vi "interfaceLoop idleStateCheck.vi"(7 "laserRefnum":refnum<vi>, 8 "error in (no error)":errorcluster, 9 "connectStateRefnum":refnum<data-value>, 11 "Stop":refnum<vi>) -> (0 "error out":errorcluster)   [LabVIEW 2018]
uses:
  PublicSubVI/Ctl/RegistyFunc.ctl
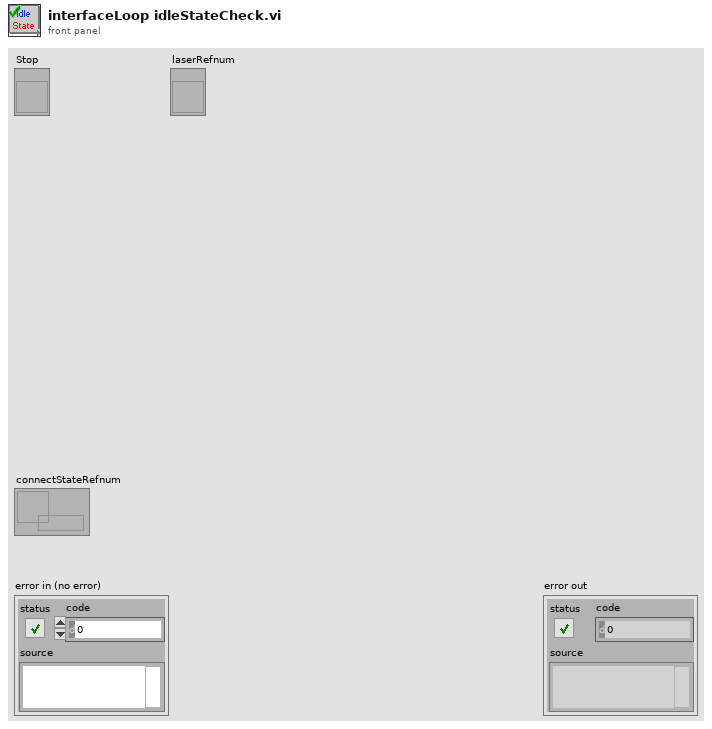
[diagram p1: front panel]
types:
  T1 = typedef "RegistyFunc.ctl" = enum16{"None", "FileAutoSave", "FileNoise", "FileSN", "ExeStatu", "WorkFolderPath", "MethodPath", "AVGItem", "LoopItem", "AutoRun", "BGColor", "LineColor", "LineWidth", "XGrid", "YGrid", "DeviceRefnum"}
  T2 = enum16{"init", "writeState", "readState", "close"}
  T3 = enum8{"Enabled", "Disabled", "Disabled and Grayed Out"}
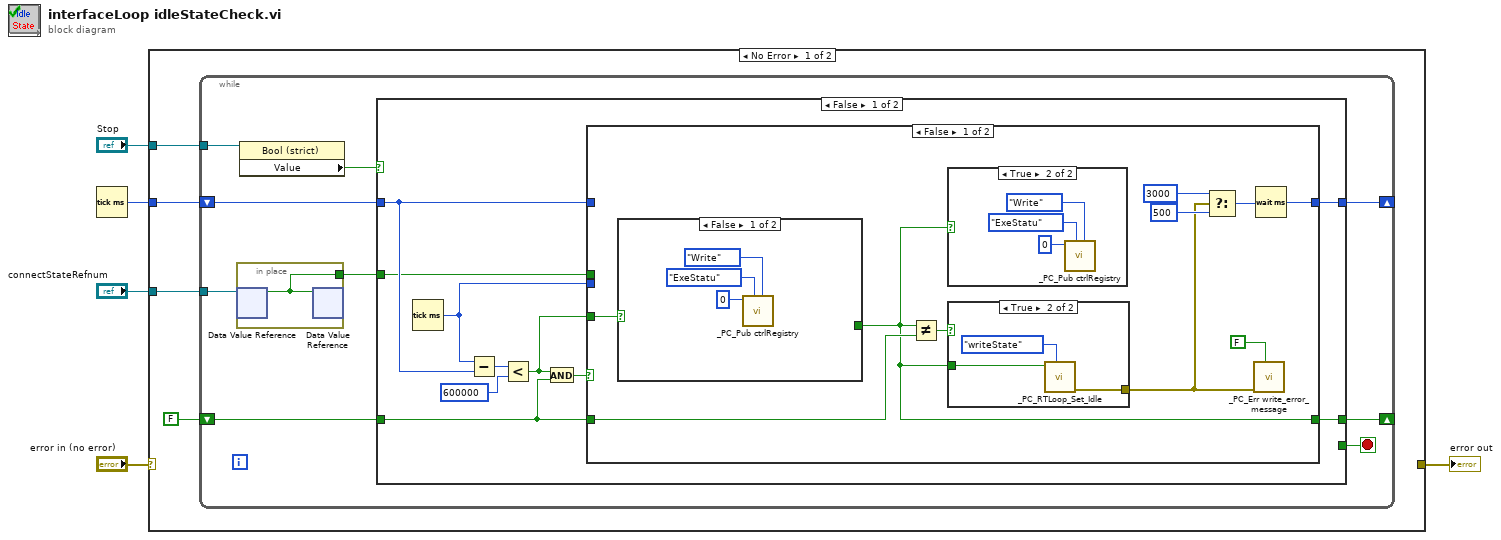
[diagram p0: block diagram]
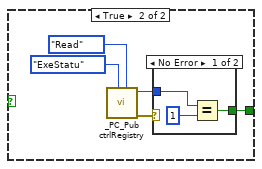
[diagram p2: hidden frame]
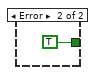
[diagram p3: hidden frame]
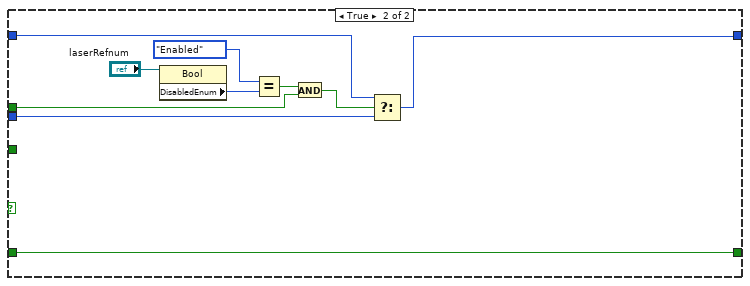
[diagram p6: hidden frame]
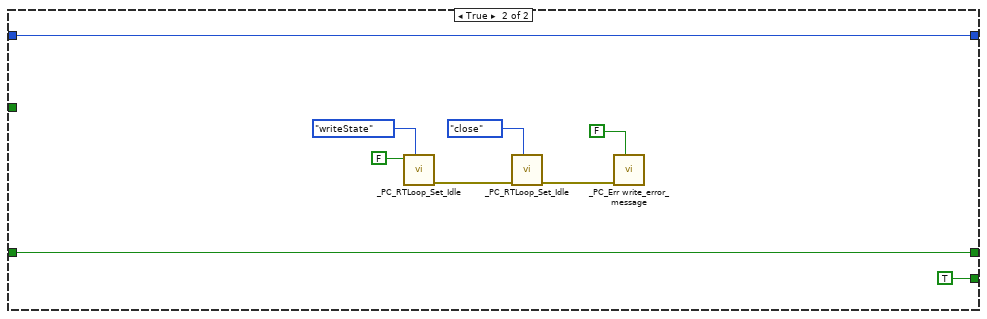
[diagram p7: hidden frame]
diagram:
  n1 = Tick Count (ms)() -> (millisecond timer value=w2:u32)
  n2 = case shown="No Error" "error in (no error)" {
    selector: "error in (no error)" -> [_ w77]
    tunnel: [_ w77] -> w4
    tunnel: "Stop" -> [w8 _]
    tunnel: w2 -> [w7 _]
    tunnel: "connectStateRefnum" -> [w6 _]
    frame No Error {
      n3 = while {
        tunnel: w8 -> [w18]
        shift-right: [w12] -> _
        shift-left: FALSE -> [w14]
        shift-right: [w13] -> _
        shift-left: w7 -> [w15]
        tunnel: w6 -> [w11]
        stop <- w16 stop-if-true
        n4 = in-place {
          in-place-border: [w19] -> w10
          n5 = in-place-dvr #1(w11) -> (w19:bool)  [unwired: 1 out]
          n6 = in-place-dvr #1(w19) -> ()  [unwired: 2 out]
        }
        n7 = property class="Bool (strict)"(reference=w18) -> ("Value"=w17:bool)  [unwired: 1 in, 2 out]
        n8 = case shown="False" w17 {
          tunnel: [_ TRUE] -> w16
          tunnel: w15 -> [w26 w75]
          tunnel: w14 -> [w24 w72]
          tunnel: [w25 w75] -> w13
          tunnel: [w23 w72] -> w12
          tunnel: w10 -> [w21 _]
          frame False {
            n9 = Tick Count (ms)() -> (millisecond timer value=w20:u32)
            n10 = Subtract(x=w20, y=w26) -> (x-y=w29:u32)
            n11 = Less?(x=w29, y=u32 600000) -> (x < y?=w22:bool)
            n12 = And(x=w22, y=w24) -> (x .and. y?=w27:bool)
            n13 = case shown="False" w27 {
              tunnel: w26 -> [_ w66]
              tunnel: [w36 w64] -> w25
              tunnel: w24 -> [w39 w67]
              tunnel: [w37 w67] -> w23
              tunnel: w22 -> [w35 _]
              tunnel: w21 -> [_ w59]
              tunnel: w20 -> [_ w65]
              frame False {
                n14 = case shown="False" w35 {
                  tunnel: [_ w43] -> w37
                  frame False {
                    n15 = call "_PC_Pub ctrlRegistry.vi"("type"=enum16{"None", "Write", "Read"}."Write", "function"=RegistyFunc."ExeStatu", "write value"=u32 0 ("y")) -> ()  [unwired: 5 in, 4 out]
                  }
                  frame True {
                    n16 = call "_PC_Pub ctrlRegistry.vi"("type"=enum16{"None", "Write", "Read"}."Read", "function"=RegistyFunc."ExeStatu") -> ("error out"=w45:errorcluster, "DWORD outpur"=w44:u32)  [unwired: 6 in, 2 out]
                    n17 = case shown="No Error" w45 {
                      tunnel: w44 -> [w50 _]
                      tunnel: [w48 TRUE] -> w43
                      frame No Error {
                        n18 = Equal?(x=w50, y=u32 1) -> (x = y?=w48:bool)
                      }
                      frame Error {
                      }
                    }
                  }
                }
                n19 = Not Equal?(x=w37, y=w39) -> (x != y?=w38:bool)
                n20 = case shown="True" w37 {
                  frame False {
                  }
                  frame True {
                    n21 = call "_PC_Pub ctrlRegistry.vi"("type"=enum16{"None", "Write", "Read"}."Write", "function"=RegistyFunc."ExeStatu", "write value"=u32 0 ("y")) -> ()  [unwired: 5 in, 4 out]
                  }
                }
                n22 = case shown="True" w38 {
                  tunnel: w37 -> [_ w57]
                  tunnel: [_ w55] -> w30
                  frame False {
                  }
                  frame True {
                    n23 = call "_PC_RTLoop_Set_Idle.vi"("Function"=T2."writeState", "exe_state"=w57) -> ("error out"=w55:errorcluster)  [unwired: 8 in, 1 out]
                  }
                }
                n24 = Select(t=u32 3000, s=w30, f=u32 500 ("milliseconds to wait")) -> (s? t:f=w32:u32)
                n25 = call "_PC_Err write_error_message.vi"("show msg( T )"=FALSE, "error in"=w30) -> ()  [unwired: 9 in, 1 out]
                n26 = Wait (ms)(milliseconds to wait=w32) -> (millisecond timer value=w36:u32)
              }
              frame True {
                n27 = property class="Bool"(reference="laserRefnum") -> ("DisabledEnum"=w61:T3)  [unwired: 1 in, 2 out]
                n28 = Equal?(x=T3."Enabled" ("y"), y=w61) -> (x = y?=w60:bool)
                n29 = And(x=w60, y=w59) -> (x .and. y?=w58:bool)
                n30 = Select(t=w66, s=w58, f=w65) -> (s? t:f=w64:u32)
              }
            }
          }
          frame True {
            n31 = call "_PC_RTLoop_Set_Idle.vi"("Function"=T2."writeState", "exe_state"=FALSE ("exe_statu")) -> ("error out"=w73:errorcluster)  [unwired: 8 in, 1 out]
            n32 = call "_PC_RTLoop_Set_Idle.vi"("Function"=T2."close", "error in (no error)"=w73) -> ("error out"=w69:errorcluster)  [unwired: 8 in, 1 out]
            n33 = call "_PC_Err write_error_message.vi"("show msg( T )"=FALSE, "error in"=w69) -> ()  [unwired: 9 in, 1 out]
          }
        }
      }
    }
    frame Error {
    }
  }
  "error out" <- w4
